vi "NMRFMTCP3.vi"() -> ()   [LabVIEW 2013]
uses:
  <vilib>/Analysis/2dsp.llb/Power Spectrum (DBL).vi
  <vilib>/Analysis/NI_AALBase.lvlib
  <vilib>/Analysis/NI_AALPro.lvlib
panel:
  out "Color Box":u32(colorbox)=16775210
  out "Measurement":enum16{"TEQ", "POL", "QCV"}(ring)
  in  "IP Address":string="192.168.0.4"
  out "FFT Vrms":dbl[](graph)=[0.015646766169154235, 0.0024982110948134676, 0.004931932619290262, 0.0008849248647205256, 0.002350996880382093, 0.0030163818070642833, 0.00321873871167239, 0.003596382576137373, 0.003663324666758867, 0.0009994820127704742, 0.0010747177604605467, 0.000922401354019206, 0.0012391697464639705, 0.0006999488109473508, 0.0009425280240178242, 0.0004953318625840751, 0.00024739643492388146, 0.00025317160361917977, 0.0006820660010904889, 0.0002670742831143547, 0.0002957484875645955, 0.00011731788024214158, 0.00015619144084108466, 7.076944387364928e-05, 0.00012524370826080074, 6.018279383692433e-05, 0.00024316035804602647, 0.00011417007815996506, 0.00010403858000381052, 4.3666360249968e-05, 8.722358525155538e-05, 6.472666110972202e-05, 7.949448204134939e-05, 4.547885976303066e-05, 3.653057660652789e-05, 9.501808066980672e-05, 2.9078658072371083e-05, 3.260626662558661e-05, 8.634700453978882e-05, 3.3459882147928455e-05, 8.341394425177981e-06, 8.711681853332232e-05, 6.11475957176423e-05, 4.284137586805631e-05, 4.7823392907281645e-06, 6.861730772494631e-05, 4.294940371852622e-05, 6.594416880768872e-05, 3.707630870344957e-05, 4.7322214771994784e-05, 8.140802356743123e-05, 4.401860468243618e-05, 6.432881992133859e-05, 7.158037542006712e-05, 5.347541272067149e-05, 1.0438009970739653e-05, 5.274129687041643e-05, 4.12553853761029e-05, 4.054935764826345e-05, 4.9349720124767846e-05, 2.4106567936024834e-05, 5.5044880104172067e-05, 6.473487682465393e-05, 1.8485431296046827e-05, 3.53153542517612e-05, 3.619008888621546e-05, 2.3642641556844984e-05, 1.9900497512436724e-05, 4.748254709029596e-05, 3.3152048109749e-05, 8.963711407032085e-06, 4.311995880312886e-05, 2.8267193875743532e-05, 1.7998716826374374e-05, 1.6139994180526443e-05, 6.40939445577451e-05, 3.5067385634575733e-05, 4.0420880711354366e-05, 2.7627165315509168e-05, 2.4593484558717827e-05, 1.625301397326756e-05, 1.58501158271677e-05, 4.3237292394627824e-05, 4.0973014105816716e-05, 2.8866404509190905e-05, 1.401615252343598e-05, 8.5877689760548e-06, 3.526207416355205e-05, 3.887541708076588e-05, 2.0945078547097e-05, 1.702451226539483e-05, 2.5281225738434016e-05, 1.5811372510805386e-05, 1.545238635589902e-05, 3.132846060147881e-05, 5.362881939741909e-05, 3.641158036427663e-05, 3.235440483664354e-05, 4.0993236124899505e-05, 3.337304052641068e-05, 5.448938806072747e-05, 5.448938806072747e-05, 3.337304052641068e-05, 4.0993236124899505e-05, 3.235440483664354e-05, 3.641158036427663e-05, 5.362881939741909e-05, 3.132846060147881e-05, 1.545238635589902e-05, 1.5811372510805386e-05, 2.5281225738434016e-05, 1.702451226539483e-05, 2.0945078547097e-05, 3.887541708076588e-05, 3.526207416355205e-05, 8.5877689760548e-06, 1.401615252343598e-05, 2.8866404509190905e-05, 4.0973014105816716e-05, 4.3237292394627824e-05, 1.58501158271677e-05, 1.625301397326756e-05, 2.4593484558717827e-05, 2.7627165315509168e-05, 4.0420880711354366e-05, 3.5067385634575733e-05, 6.40939445577451e-05, 1.6139994180526443e-05, 1.7998716826374374e-05, 2.8267193875743532e-05, 4.311995880312886e-05, 8.963711407032085e-06, 3.3152048109749e-05, 4.748254709029596e-05, 1.9900497512436724e-05, 2.3642641556844984e-05, 3.619008888621546e-05, 3.53153542517612e-05, 1.8485431296046827e-05, 6.473487682465393e-05, 5.5044880104172067e-05, 2.4106567936024834e-05, 4.9349720124767846e-05, 4.054935764826345e-05, 4.12553853761029e-05, 5.274129687041643e-05, 1.0438009970739653e-05, 5.347541272067149e-05, 7.158037542006712e-05, 6.432881992133859e-05, 4.401860468243618e-05, 8.140802356743123e-05, 4.7322214771994784e-05, 3.707630870344957e-05, 6.594416880768872e-05, 4.294940371852622e-05, 6.861730772494631e-05, 4.7823392907281645e-06, 4.284137586805631e-05, 6.11475957176423e-05, 8.711681853332232e-05, 8.341394425177981e-06, 3.3459882147928455e-05, 8.634700453978882e-05, 3.260626662558661e-05, 2.9078658072371083e-05, 9.501808066980672e-05, 3.653057660652789e-05, 4.547885976303066e-05, 7.949448204134939e-05, 6.472666110972202e-05, 8.722358525155538e-05, 4.3666360249968e-05, 0.00010403858000381052, 0.00011417007815996506, 0.00024316035804602647, 6.018279383692433e-05, 0.00012524370826080074, 7.076944387364928e-05, 0.00015619144084108466, 0.00011731788024214158, 0.0002957484875645955, 0.0002670742831143547, 0.0006820660010904889, 0.00025317160361917977, 0.00024739643492388146, 0.0004953318625840751, 0.0009425280240178242, 0.0006999488109473508, 0.0012391697464639705, 0.000922401354019206, 0.0010747177604605467, 0.0009994820127704742, 0.003663324666758867, 0.003596382576137373, 0.00321873871167239, 0.0030163818070642833, 0.002350996880382093, 0.0008849248647205256, 0.004931932619290262, 0.0024982110948134676]
  out "Raw NMR Graph / Ave":cluster{dbl, "Step Width (MHz)":dbl, dbl[][]}(graph)={212.47, "Step Width (MHz)"=0.0025, [[0.032, 0.031, 0.031, 0.031, 0.03, 0.03, 0.029, 0.029, 0.027, 0.027, 0.026, 0.025, 0.024, 0.023, 0.023, 0.023, 0.022, 0.021, 0.021, 0.021, 0.02, 0.02, 0.02, 0.019, 0.018, 0.017, 0.017, 0.016, 0.016, 0.015, 0.014, 0.014, 0.013, 0.013, 0.012, 0.012, 0.011, 0.011, 0.01, 0.009, 0.009, 0.009, 0.008, 0.008, 0.007, 0.007, 0.006, 0.006, 0.005, 0.005, 0.005, 0.005, 0.005, 0.004, 0.004, 0.004, 0.004, 0.003, 0.003, 0.002, 0.002, 0.002, 0.002, 0.002, 0.001, 0.0, 0.001, 0.001, -0.0, -0.0, -0.0, 0.0, 0.0, -0.0, -0.0, -0.0, -0.001, -0.0, -0.0, -0.0, -0.0, -0.0, 0.0, 0.001, 0.003, 0.004, 0.005, 0.007, 0.009, 0.011, 0.013, 0.016, 0.021, 0.026, 0.032, 0.039, 0.047, 0.054, 0.06, 0.061, 0.059, 0.054, 0.047, 0.038, 0.03, 0.023, 0.019, 0.015, 0.011, 0.008, 0.006, 0.005, 0.004, 0.003, 0.003, 0.003, 0.003, 0.003, 0.004, 0.006, 0.008, 0.01, 0.013, 0.016, 0.02, 0.025, 0.031, 0.037, 0.043, 0.047, 0.049, 0.049, 0.045, 0.038, 0.032, 0.026, 0.021, 0.016, 0.013, 0.009, 0.007, 0.006, 0.005, 0.004, 0.005, 0.005, 0.007, 0.009, 0.01, 0.013, 0.017, 0.021, 0.024, 0.026, 0.027, 0.026, 0.023, 0.02, 0.016, 0.013, 0.01, 0.008, 0.005, 0.004, 0.003, 0.003, 0.003, 0.003, 0.004, 0.005, 0.006, 0.008, 0.01, 0.013, 0.016, 0.018, 0.021, 0.022, 0.023, 0.023, 0.022, 0.021, 0.02, 0.019, 0.019, 0.017, 0.016, 0.014, 0.013, 0.012, 0.012, 0.012, 0.013, 0.014, 0.015, 0.018, 0.022, 0.026, 0.03, 0.035, 0.04], [0.03140634920634919, 0.03086031746031746, 0.030584126984126957, 0.0301301587301587, 0.029622222222222175, 0.029066666666666595, 0.028504761904761852, 0.027974603174603135, 0.02739047619047618, 0.0268095238095238, 0.026231746031746002, 0.02564126984126982, 0.025031746031746002, 0.02441269841269838, 0.023882539682539648, 0.023307936507936475, 0.0227269841269841, 0.02213650793650791, 0.021523809523809483, 0.020942857142857096, 0.020365079365079333, 0.01980317460317458, 0.019266666666666633, 0.018736507936507895, 0.01819047619047616, 0.01759682539682536, 0.01702857142857139, 0.016403174603174562, 0.015853968253968235, 0.015317460317460296, 0.014796825396825364, 0.014266666666666619, 0.013739682539682496, 0.013152380952380915, 0.012609523809523782, 0.012111111111111081, 0.011660317460317435, 0.011161904761904729, 0.010619047619047589, 0.010193650793650765, 0.00968888888888886, 0.009247619047619022, 0.008771428571428543, 0.008253968253968225, 0.007936507936507912, 0.00743174603174601, 0.006990476190476172, 0.006542857142857125, 0.0061142857142856945, 0.005711111111111095, 0.005276190476190463, 0.004882539682539673, 0.004539682539682529, 0.004184126984126974, 0.0038126984126984078, 0.0034603174603174613, 0.003066666666666669, 0.0027301587301587324, 0.002390476190476192, 0.0021015873015873027, 0.0017650793650793664, 0.0014476190476190485, 0.0011492063492063499, 0.0009174603174603177, 0.0007047619047619049, 0.0004952380952380952, 0.00022857142857142857, 3.1746031746029874e-06, -0.00013333333333333353, -0.00031428571428571454, -0.0004984126984126985, -0.000612698412698413, -0.0006952380952380956, -0.0007269841269841271, -0.0007746031746031748, -0.000758730158730159, -0.0006634920634920635, -0.0005492063492063494, -0.00037460317460317474, -0.0001333333333333334, 0.00021587301587301584, 0.0006126984126984127, 0.001111111111111112, 0.0017841269841269854, 0.002574603174603176, 0.0035968253968253947, 0.0047682539682539615, 0.006317460317460301, 0.00816507936507934, 0.010574603174603145, 0.013438095238095197, 0.016961904761904737, 0.021368253968253936, 0.026517460317460318, 0.032958730158730166, 0.03983174603174603, 0.0473174603174603, 0.054425396825396766, 0.059574603174603134, 0.06149523809523812, 0.05948253968253961, 0.053911111111111056, 0.046282539682539675, 0.037920634920634896, 0.03019682539682538, 0.023441269841269805, 0.018063492063492025, 0.01379047619047615, 0.010320634920634897, 0.007819047619047595, 0.005866666666666651, 0.004488888888888881, 0.0035650793650793653, 0.0029047619047619065, 0.0026444444444444462, 0.002625396825396827, 0.002949206349206351, 0.0036476190476190454, 0.004552380952380944, 0.0059238095238095066, 0.00776507936507934, 0.010101587301587271, 0.012961904761904728, 0.016565079365079338, 0.020765079365079327, 0.025907936507936477, 0.031787301587301545, 0.037806349206349205, 0.043555555555555535, 0.04799365079365076, 0.0500857142857143, 0.049082539682539665, 0.045193650793650765, 0.03926984126984125, 0.03255238095238093, 0.025993650793650763, 0.02026984126984124, 0.015615873015872984, 0.012006349206349177, 0.009222222222222194, 0.007247619047619024, 0.005873015873015858, 0.005019047619047606, 0.00465396825396824, 0.0048190476190476065, 0.005355555555555541, 0.006539682539682519, 0.008352380952380924, 0.010666666666666637, 0.013707936507936476, 0.016990476190476167, 0.020568253968253937, 0.02367936507936505, 0.02587619047619045, 0.026533333333333294, 0.02548888888888887, 0.022977777777777767, 0.019488888888888865, 0.015676190476190444, 0.012015873015872985, 0.008888888888888863, 0.0064412698412698215, 0.004644444444444433, 0.0033936507936507955, 0.0026476190476190493, 0.0023269841269841283, 0.0023682539682539695, 0.0027968253968253987, 0.0034666666666666682, 0.004488888888888881, 0.005847619047619032, 0.007587301587301563, 0.00974285714285711, 0.01238412698412695, 0.015180952380952366, 0.017987301587301552, 0.020568253968253947, 0.022244444444444414, 0.02298412698412696, 0.022806349206349177, 0.021958730158730122, 0.020914285714285673, 0.01988253968253965, 0.018968253968253926, 0.018088888888888863, 0.01697142857142854, 0.015765079365079336, 0.014476190476190452, 0.013276190476190433, 0.012355555555555535, 0.011892063492063456, 0.011822222222222185, 0.012349206349206322, 0.013492063492063461, 0.015085714285714256, 0.017514285714285687, 0.020606349206349173, 0.02439365079365076, 0.028895238095238068, 0.033825396825396835, 0.03893333333333329]]}
  in  "GPIB Addr (28)":refnum<visa-resource-name>="GPIB0::28::INSTR"
  out "Pedestal (V)":dbl=-0.0019038541666667472 format="%_2g"
  in  "Open Global Panel":bool=TRUE
  out "Peak center (MHz)":sgl=212.71716 format="%.3f"
  out "Telnet error out":errorcluster
  out "+3.3V supply":dbl=3.279 format="%_4g"
  out "Temp (C)":dbl=30.5 format="%_4g"
  out "RF OK":bool=TRUE
  out "Peak area (V-MHz)":sgl=3.3110082 format="%.5f"
  out "NMR Graph + Fit":cluster{cluster{dbl, "Numeric":dbl}[]}[](graph)=[{[{212.47, "Numeric"=0.0010780416666670367}, {212.4725, "Numeric"=0.0007280416666664439}, {212.475, "Numeric"=0.0013715416666658662}, {212.4775, "Numeric"=0.0020085416666652993}, {212.48, "Numeric"=0.001639041666664739}, {212.4825, "Numeric"=0.0022630416666642008}, {212.48499999999999, "Numeric"=0.001880541666663669}, {212.4875, "Numeric"=0.0024915416666700567}, {212.49, "Numeric"=0.001096041666669473}, {212.4925, "Numeric"=0.0016940416666689053}, {212.495, "Numeric"=0.001285541666668344}, {212.4975, "Numeric"=0.0008705416666678007}, {212.5, "Numeric"=0.00044904166666726465}, {212.5025, "Numeric"=2.1041666666739463e-05}, {212.505, "Numeric"=0.0005865416666662295}, {212.5075, "Numeric"=0.0011455416666657304}, {212.51, "Numeric"=0.0006980416666652412}, {212.5125, "Numeric"=0.0002440416666647698}, {212.515, "Numeric"=0.0007835416666643032}, {212.5175, "Numeric"=0.0013165416666698774}, {212.52, "Numeric"=0.0008430416666693587}, {212.5225, "Numeric"=0.0013630416666688587}, {212.525, "Numeric"=0.0018765416666683661}, {212.5275, "Numeric"=0.001383541666667887}, {212.53, "Numeric"=0.0008840416666674187}, {212.5325, "Numeric"=0.0003780416666669681}, {212.535, "Numeric"=0.0008655416666665259}, {212.5375, "Numeric"=0.0003465416666660901}, {212.54, "Numeric"=0.000821041666665673}, {212.5425, "Numeric"=0.00028904166666526235}, {212.545, "Numeric"=-0.0002494583333351322}, {212.54749999999999, "Numeric"=0.00020554166666448322}, {212.55, "Numeric"=-0.0003459583333308277}, {212.5525, "Numeric"=9.604166666873828e-05}, {212.555, "Numeric"=-0.000468458333331684}, {212.5575, "Numeric"=-3.945833333209459e-05}, {212.56, "Numeric"=-0.0006169583333324952}, {212.5625, "Numeric"=-0.0002009583333328806}, {212.565, "Numeric"=-0.0007914583333332561}, {212.5675, "Numeric"=-0.0013884583333336207}, {212.57, "Numeric"=-0.0009919583333339718}, {212.5725, "Numeric"=-0.0006019583333343103}, {212.575, "Numeric"=-0.001218458333334639}, {212.5775, "Numeric"=-0.000841458333334954}, {212.58, "Numeric"=-0.0014709583333310846}, {212.5825, "Numeric"=-0.0011069583333314509}, {212.585, "Numeric"=-0.0017494583333318063}, {212.5875, "Numeric"=-0.0013984583333321475}, {212.59, "Numeric"=-0.0020539583333324795}, {212.5925, "Numeric"=-0.0017159583333327972}, {212.595, "Numeric"=-0.0013844583333331058}, {212.5975, "Numeric"=-0.0010594583333334}, {212.6, "Numeric"=-0.0007409583333336843}, {212.6025, "Numeric"=-0.001428958333333957}, {212.605, "Numeric"=-0.001123458333334217}, {212.6075, "Numeric"=-0.0008244583333344643}, {212.60999999999999, "Numeric"=-0.0005319583333347018}, {212.6125, "Numeric"=-0.0012459583333317113}, {212.615, "Numeric"=-0.0009664583333319982}, {212.6175, "Numeric"=-0.0016934583333322725}, {212.62, "Numeric"=-0.001426958333332536}, {212.6225, "Numeric"=-0.0011669583333327868}, {212.625, "Numeric"=-0.0009134583333330268}, {212.6275, "Numeric"=-0.0006664583333332542}, {212.63, "Numeric"=-0.00142595833333347}, {212.6325, "Numeric"=-0.002191958333333673}, {212.635, "Numeric"=-0.0009644583333338654}, {212.6375, "Numeric"=-0.0007434583333340459}, {212.64, "Numeric"=-0.0015289583333342144}, {212.6425, "Numeric"=-0.001320958333332043}, {212.645, "Numeric"=-0.0011194583333322622}, {212.6475, "Numeric"=-0.0009244583333324688}, {212.65, "Numeric"=-0.0007359583333326637}, {212.6525, "Numeric"=-0.0005539583333328468}, {212.655, "Numeric"=-0.0003784583333330182}, {212.6575, "Numeric"=-0.00020945833333317794}, {212.66, "Numeric"=-0.001046958333333326}, {212.6625, "Numeric"=0.0001090416666665382}, {212.665, "Numeric"=0.0002585416666664143}, {212.6675, "Numeric"=0.0004015416666663021}, {212.67, "Numeric"=0.0005380416666662016}, {212.67249999999999, "Numeric"=0.0006680416666661128}, {212.675, "Numeric"=0.0007915416666674031}, {212.6775, "Numeric"=0.0019085416666672643}, {212.68, "Numeric"=0.004019041666667137}, {212.6825, "Numeric"=0.005123041666667022}, {212.685, "Numeric"=0.006220541666666918}, {212.6875, "Numeric"=0.008311541666666828}, {212.69, "Numeric"=0.010396041666666748}, {212.6925, "Numeric"=0.012474041666666678}, {212.695, "Numeric"=0.014545541666666623}, {212.6975, "Numeric"=0.017610541666666576}, {212.7, "Numeric"=0.022669041666666546}, {212.7025, "Numeric"=0.027721041666666522}, {212.705, "Numeric"=0.033766541666666997}, {212.7075, "Numeric"=0.040805541666666924}, {212.71, "Numeric"=0.048838041666666866}, {212.7125, "Numeric"=0.055864041666666815}, {212.715, "Numeric"=0.061883541666666785}, {212.7175, "Numeric"=0.06289654166666676}, {212.72, "Numeric"=0.06090304166666675}, {212.7225, "Numeric"=0.05590304166666675}, {212.725, "Numeric"=0.04889654166666676}, {212.7275, "Numeric"=0.039883541666666786}, {212.73, "Numeric"=0.03186404166666682}, {212.7325, "Numeric"=0.024838041666666866}, {212.73499999999999, "Numeric"=0.020805541666666923}, {212.7375, "Numeric"=0.016766541666666517}, {212.74, "Numeric"=0.012721041666666526}, {212.7425, "Numeric"=0.009669041666666546}, {212.745, "Numeric"=0.007610541666666579}, {212.7475, "Numeric"=0.006545541666666623}, {212.75, "Numeric"=0.005474041666666679}, {212.7525, "Numeric"=0.004396041666666748}, {212.755, "Numeric"=0.004311541666666827}, {212.7575, "Numeric"=0.004220541666666919}, {212.76, "Numeric"=0.004123041666667022}, {212.7625, "Numeric"=0.004019041666667137}, {212.765, "Numeric"=0.004908541666667265}, {212.7675, "Numeric"=0.006791541666666036}, {212.77, "Numeric"=0.008668041666666113}, {212.7725, "Numeric"=0.010538041666666203}, {212.775, "Numeric"=0.013401541666666301}, {212.7775, "Numeric"=0.016258541666666414}, {212.78, "Numeric"=0.02010904166666654}, {212.7825, "Numeric"=0.024953041666666675}, {212.785, "Numeric"=0.03079054166666682}, {212.7875, "Numeric"=0.03662154166666698}, {212.79, "Numeric"=0.04244604166666715}, {212.7925, "Numeric"=0.04626404166666734}, {212.795, "Numeric"=0.04807554166666753}, {212.79749999999999, "Numeric"=0.04788054166666774}, {212.8, "Numeric"=0.04367904166666563}, {212.8025, "Numeric"=0.03647104166666578}, {212.805, "Numeric"=0.030256541666665953}, {212.8075, "Numeric"=0.024035541666666133}, {212.81, "Numeric"=0.018808041666666327}, {212.8125, "Numeric"=0.01357404166666653}, {212.815, "Numeric"=0.010333541666666744}, {212.8175, "Numeric"=0.0060865416666669725}, {212.82, "Numeric"=0.0038330416666672133}, {212.8225, "Numeric"=0.002573041666667464}, {212.825, "Numeric"=0.0013065416666677276}, {212.8275, "Numeric"=3.354166666800183e-05}, {212.83, "Numeric"=0.0007540416666650743}, {212.8325, "Numeric"=0.00046804166666529826}, {212.835, "Numeric"=0.0021755416666655357}, {212.8375, "Numeric"=0.0038765416666657823}, {212.84, "Numeric"=0.004571041666666043}, {212.8425, "Numeric"=0.007259041666666315}, {212.845, "Numeric"=0.010940541666666602}, {212.8475, "Numeric"=0.014615541666666895}, {212.85, "Numeric"=0.017284041666667204}, {212.8525, "Numeric"=0.018946041666667517}, {212.855, "Numeric"=0.019601541666667853}, {212.8575, "Numeric"=0.01825054166666819}, {212.85999999999999, "Numeric"=0.01489304166666855}, {212.8625, "Numeric"=0.011529041666664741}, {212.865, "Numeric"=0.007158541666665046}, {212.8675, "Numeric"=0.0037815416666653603}, {212.87, "Numeric"=0.00039804166666569055}, {212.8725, "Numeric"=-0.001991958333333971}, {212.875, "Numeric"=-0.00538845833333362}, {212.8775, "Numeric"=-0.006791458333333256}, {212.88, "Numeric"=-0.00820095833333288}, {212.8825, "Numeric"=-0.008616958333332495}, {212.885, "Numeric"=-0.009039458333332095}, {212.8875, "Numeric"=-0.009468458333331684}, {212.89, "Numeric"=-0.008903958333331262}, {212.8925, "Numeric"=-0.00834595833333589}, {212.895, "Numeric"=-0.007794458333335517}, {212.8975, "Numeric"=-0.006249458333335132}, {212.9, "Numeric"=-0.004710958333334737}, {212.9025, "Numeric"=-0.002178958333334328}, {212.905, "Numeric"=0.0003465416666660901}, {212.9075, "Numeric"=0.0018655416666665233}, {212.91, "Numeric"=0.004378041666666968}, {212.9125, "Numeric"=0.004884041666667419}, {212.915, "Numeric"=0.005383541666667887}, {212.9175, "Numeric"=0.004876541666668365}, {212.92, "Numeric"=0.003363041666668857}, {212.92249999999999, "Numeric"=0.0018430416666693596}, {212.925, "Numeric"=0.00031654166666385004}, {212.9275, "Numeric"=-0.0012164583333356986}, {212.93, "Numeric"=-0.001755958333335232}, {212.9325, "Numeric"=-0.004301958333334756}, {212.935, "Numeric"=-0.005854458333334269}, {212.9375, "Numeric"=-0.008413458333333769}, {212.94, "Numeric"=-0.00997895833333326}, {212.9425, "Numeric"=-0.011550958333332736}, {212.945, "Numeric"=-0.012129458333332201}, {212.9475, "Numeric"=-0.012714458333331655}, {212.95, "Numeric"=-0.012305958333331094}, {212.9525, "Numeric"=-0.011903958333330526}, {212.955, "Numeric"=-0.011508458333336854}, {212.9575, "Numeric"=-0.009119458333336335}, {212.96, "Numeric"=-0.005736958333335799}, {212.9625, "Numeric"=-0.002360958333335261}, {212.965, "Numeric"=0.0010085416666652984}, {212.9675, "Numeric"=0.00537154166666587}, {212.97, "Numeric"=0.009728041666666444}]}]
  out "# Good Spectra":i32=989
  out "Pedestal OK":bool=TRUE
  out "Sweep #":i32=316
  out "1st Sweep":bool
  out "ADC volts OK":bool=TRUE
  out "Peak Height Distribution":cluster{"Y":dbl[], "Y":dbl[]}[](graph)=[{"Y"=[0.06173175000000009, 0.061768833333333426, 0.06180591666666676, 0.06184300000000009, 0.061880083333333426, 0.06191716666666676, 0.06195425000000009, 0.061991333333333426, 0.06202841666666676, 0.06206550000000009, 0.062102583333333426, 0.06213966666666676, 0.06217675000000009, 0.062213833333333426, 0.06225091666666676, 0.06228800000000009, 0.06232508333333343, 0.06236216666666676, 0.062399250000000094, 0.06243633333333343, 0.06247341666666676, 0.0625105000000001, 0.06254758333333343, 0.06258466666666676, 0.0626217500000001, 0.06265883333333343, 0.06269591666666677, 0.0627330000000001, 0.06277008333333343, 0.06280716666666676, 0.0628442500000001, 0.06288133333333343, 0.06291841666666677, 0.0629555000000001, 0.06299258333333344, 0.06302966666666676, 0.0630667500000001, 0.06310383333333343, 0.06314091666666677, 0.0631780000000001, 0.06321508333333344, 0.06325216666666676, 0.0632892500000001, 0.06332633333333343, 0.06336341666666677, 0.0634005000000001, 0.06343758333333344, 0.06347466666666676, 0.0635117500000001, 0.06354883333333343, 0.06358591666666677, 0.0636230000000001, 0.06366008333333342, 0.06369716666666676, 0.06373425000000009, 0.06377133333333343, 0.06380841666666676, 0.0638455000000001, 0.06388258333333342, 0.06391966666666676, 0.06395675000000009, 0.06399383333333343, 0.06403091666666676, 0.0640680000000001, 0.06410508333333342, 0.06414216666666676, 0.06417925000000009, 0.06421633333333343, 0.06425341666666676, 0.0642905000000001, 0.06432758333333342, 0.06436466666666676, 0.06440175000000009, 0.06443883333333343, 0.06447591666666676, 0.0645130000000001, 0.06455008333333342, 0.06458716666666676, 0.06462425000000009, 0.06466133333333343, 0.06469841666666676, 0.0647355000000001, 0.06477258333333342, 0.06480966666666677, 0.06484675000000009, 0.06488383333333343, 0.06492091666666676, 0.0649580000000001, 0.06499508333333343, 0.06503216666666677, 0.06506925000000009, 0.06510633333333343, 0.06514341666666676, 0.0651805000000001, 0.06521758333333343, 0.06525466666666677, 0.06529175000000009, 0.06532883333333343, 0.06536591666666676, 0.0654030000000001], "Y"=[1.0, 0.0, 1.0, 2.0, 2.0, 3.0, 2.0, 0.0, 3.0, 4.0, 2.0, 8.0, 6.0, 8.0, 2.0, 6.0, 4.0, 4.0, 5.0, 9.0, 6.0, 8.0, 10.0, 8.0, 7.0, 8.0, 12.0, 10.0, 10.0, 16.0, 10.0, 18.0, 13.0, 6.0, 15.0, 17.0, 17.0, 16.0, 17.0, 14.0, 19.0, 17.0, 13.0, 16.0, 23.0, 22.0, 22.0, 16.0, 26.0, 21.0, 24.0, 17.0, 19.0, 18.0, 13.0, 24.0, 18.0, 18.0, 22.0, 17.0, 17.0, 8.0, 14.0, 14.0, 14.0, 11.0, 18.0, 22.0, 16.0, 10.0, 15.0, 16.0, 8.0, 10.0, 15.0, 9.0, 3.0, 4.0, 6.0, 8.0, 7.0, 5.0, 7.0, 3.0, 6.0, 4.0, 5.0, 4.0, 4.0, 0.0, 2.0, 0.0, 1.0, 1.0, 0.0, 2.0, 1.0, 2.0, 1.0, 1.0]}]
  out "S/N":dbl=88.94507757693563 format="%_3g"
  out "Peak mean (V)":dbl=0.06354517665149992 format="%_4g"
  out "Pedestal Diff (V)":sgl=-0.00015841666 format="%.3f"
  out "Peak amp (V)":sgl=0.06289654 format="%.3f"
  out "SMT error out":errorcluster
  out "Peak RMS (mV)":dbl=0.7144316288502269 format="%.3f"
  # "E1039 NMR Panel"
  # "Results"
  # "A\nv\ne\nr\na\ng\ne\ns"
  # "S\nw\ne\ne\np"
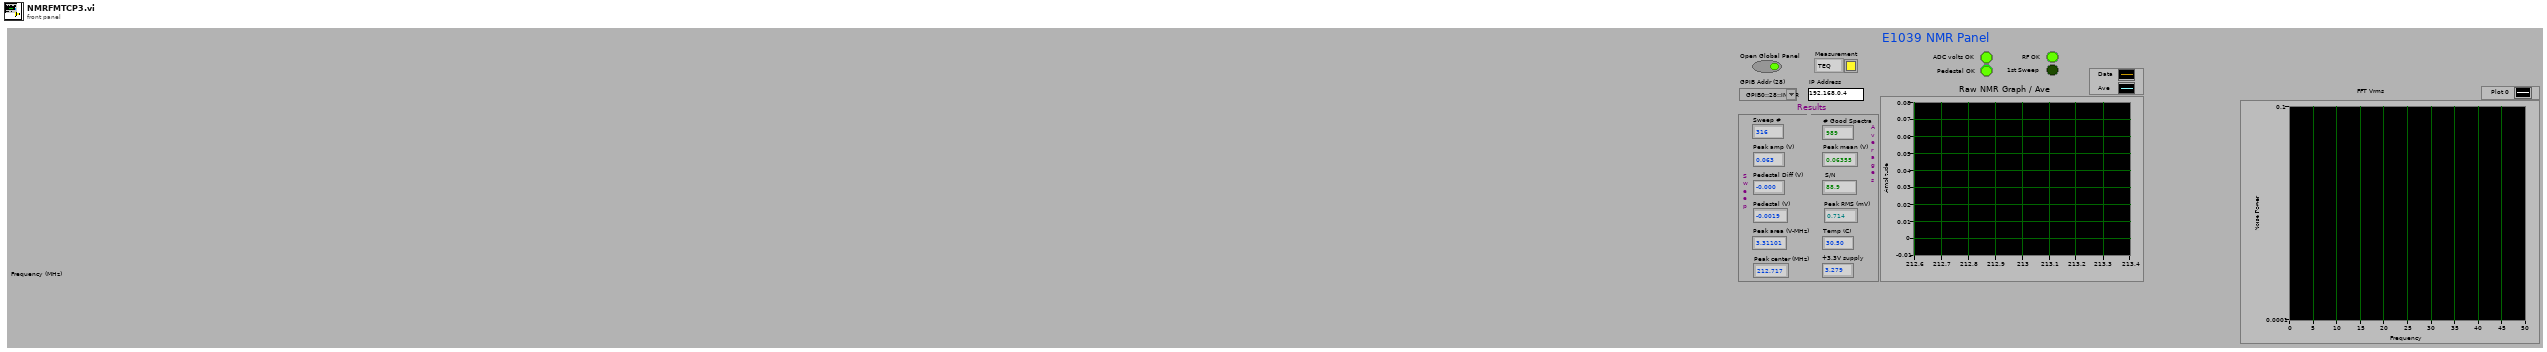
[diagram p1: front panel]
types:
  T1 = enum32{"Invalid", "Standard", "Closed", "Hidden", "Minimized", "Maximized"}
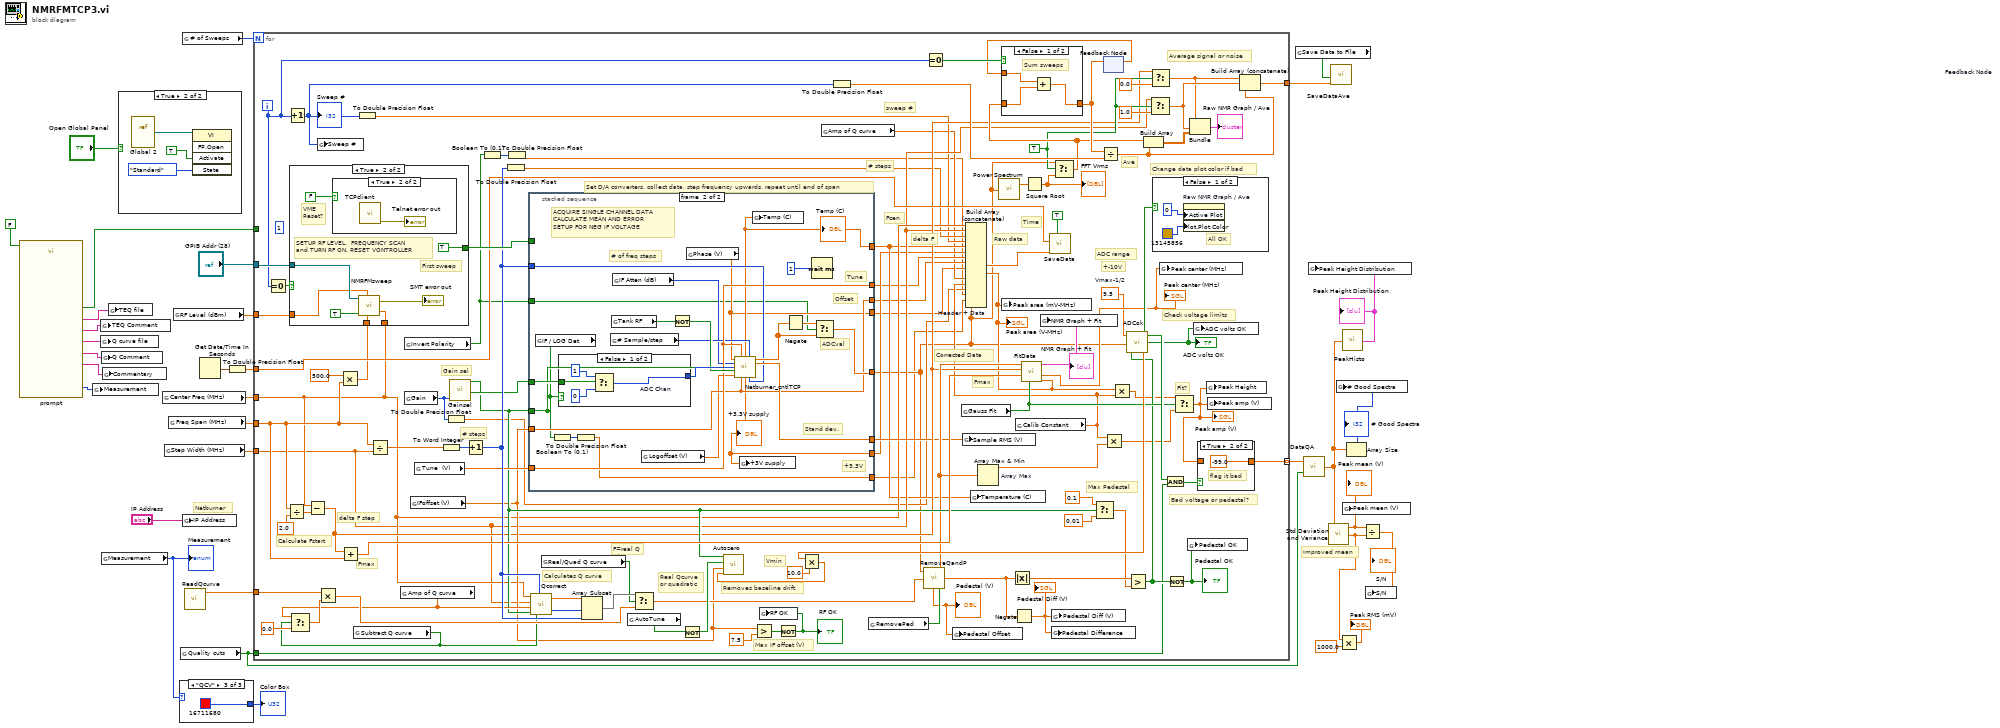
[diagram p0: block diagram]
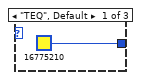
[diagram p2: hidden frame]
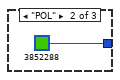
[diagram p3: hidden frame]
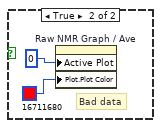
[diagram p6: hidden frame]
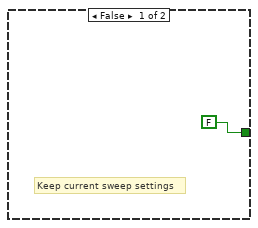
[diagram p8: hidden frame]
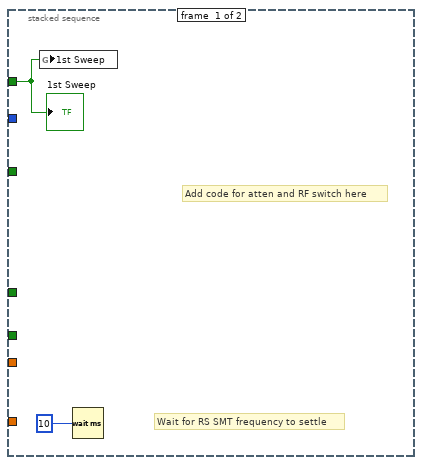
[diagram p10: hidden frame]
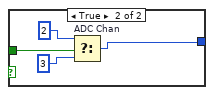
[diagram p11: hidden frame]
diagram:
  # "Netburner"
  # "Improved mean"
  n1 = call "prompt.vi"("Enable"=FALSE) -> ("Measurement"=w2:enum16{"TEQ", "POL", "QCV"}, "Run comment"=w3:string, "Q curve comment"=w4:string, "Q curve file"=w5:string, "TE Comment"=w6:string, "TE peak file"=w7:string, "OK"=w8:bool)  [unwired: 11 in, 1 out]
  n2 = global write "Global 2.vi" "Measurement"(w2) -> ()
  n3 = global write "Global 2.vi" "TEQ Comment"(w6) -> ()
  n4 = global write "Global 2.vi" "Q curve file"(w5) -> ()
  n5 = global write "Global 2.vi" "Q Comment"(w4) -> ()
  n6 = global read "Global 2.vi" "Measurement"() -> (w10:enum16{"TEQ", "POL", "QCV"})
  "Measurement" <- w10
  n7 = global write "Global 2.vi" "Commentary"(w3) -> ()
  n8 = global write "Global 2.vi" "TEQ file"(w7) -> ()
  n9 = case shown="True" "Open Global Panel" {
    frame False {
    }
    frame True {
      n10 = vi-ref "Global 2.vi"() -> (w36:refnum<vi>)
      n11 = invoke class="VI" method="FP.Open"(reference=w36, "Activate"=TRUE, "State"=T1."Standard") -> ()  [unwired: 2 in, 5 out]
    }
  }
  n12 = global read "Global 2.vi" "Center Freq (MHz)"() -> (w28:dbl)
  n13 = global read "Global 2.vi" "Step Width (MHz)"() -> (w26:dbl)
  n14 = global read "Global 2.vi" "Freq Span (MHz)"() -> (w27:dbl)
  n15 = global read "Global 2.vi" "RF Level (dBm)"() -> (w29:dbl)
  n16 = case shown="\"QCV\"" w10 {
    tunnel: [u32 16775210 ("Color Box 2") u32 3852288 ("Color Box 2") u32 16711680 ("Color Box 2")] -> w9
    frame "TEQ", Default {
    }
    frame "POL" {
    }
    frame "QCV" {
    }
  }
  "Color Box" <- w9
  n17 = global read "Global 2.vi" "Quality cuts"() -> (w25:bool)
  n18 = global write "Global 2.vi" "IP Address"("IP Address") -> ()
  n19 = global read "Global 2.vi" "# of Sweeps"() -> (w30:i32)
  n20 = call "ReadQcurve.vi"() -> ("Array"=w15:dbl[])  [unwired: 2 in]
  n21 = Get Date/Time In Seconds() -> (seconds since 1Jan1904=w31:timestamp)
  n22 = To Double Precision Float(number=w31) -> (double precision float=w16:dbl)
  n23 = for {
    N: w30 -> [_]
    tunnel: [w133] -> w33 mode=indexing
    tunnel: w25 -> [w93]
    tunnel: w28 -> [w61]
    tunnel: w27 -> [w74]
    tunnel: w26 -> [w60]
    tunnel: "GPIB Addr (28)" -> [w128]
    tunnel: w29 -> [w127]
    tunnel: w16 -> [w126]
    tunnel: w15 -> [w118]
    tunnel: [w80] -> w18
    tunnel: w8 -> [_]
    i -> [w76]
    (unwired) 1
    w66 = TRUE
    w87 = 9.5  # Vmax-1/2
    # "Average signal or noise"
    # "Check voltage limits"
    # "Ave"
    # "Max Pedestal"
    # "Gain sel"
    # "F=real Q"
    # "Real Qcurve\nor quadratic"
    # "+-10V"
    # "Change data plot color if bad"
    # "Max IF offset (V)"
    # "Fmax"
    # "Fit?"
    # "Fmax"
    # "Time"
    # "Vmin"
    # "Raw data"
    # "Corrected Data"
    # "Fcen"
    # "delta F"
    # "# steps"
    # "ADC range"
    # "sweep #"
    # "Set D/A converters, collect data, step frequency upwards, repeat until end of span"
    # "Calculates Q curve"
    # "Removes baseline drift"
    # "Bad voltage or pedestal?"
    # "# steps"
    # "Calculate Fstart"
    # "delta F step"
    n24 = Equal To 0?(x=w76) -> (x = 0?=w135:bool)
    n25 = Divide(x=w74, y=sgl 2.0) -> (x/y=w139:dbl)
    n26 = Increment(x=w76) -> (x+1=w91:i32)
    "Sweep #" <- w91
    n27 = Subtract(x=w61, y=w139) -> (x-y=w64:dbl)
    n28 = global write "Global 2.vi" "Sweep #"(w91) -> ()
    n29 = Multiply(x=500.0, y=w74) -> (x*y=w73:dbl)
    n30 = case shown="True" w135 {
      tunnel: w61 -> [_ w159]
      tunnel: w73 -> [_ w160]
      tunnel: [FALSE TRUE] -> w134
      tunnel: w128 -> [_ w156]
      tunnel: w127 -> [_ w155]
      frame False {
        # "Keep current sweep settings"
      }
      frame True {
        # "VME\nReset?"
        # "First sweep"
        # "SETUP RF LEVEL,  FREQUENCY SCAN\nand TURN RF ON. RESET VONTROLLER"
        n31 = case shown="True" FALSE {
          frame False {
          }
          frame True {
            n32 = call "TCPclient.vi"() -> ("Telnet error"=→"Telnet error out":errorcluster)  [unwired: 4 in, 3 out]
          }
        }
        n33 = call "NMRFMsweep.vi"("Center Freq (MHz)"=w159, "Freq Span (kHz)"=w160, "RF Level (dBm)"=w155, "Program"=TRUE, "GPIB Addr (28)"=w156) -> ("error out"=→"SMT error out":errorcluster)  [unwired: 2 in]
      }
    }
    n34 = Add(x=w64, y=w74) -> (x+y=w123:dbl)
    n35 = global read "Global 2.vi" "Subtract Q curve"() -> (w109:bool)
    n36 = To Double Precision Float(number=w91) -> (double precision float=w58:dbl)
    n37 = Divide(x=w74, y=w60) -> (x/y=w141:dbl)
    n38 = global read "Global 2.vi" "Amp of Q curve"() -> (w110:dbl)
    n39 = Select(t=w110, s=w109, f=0.0) -> (s? t:f=w115:dbl)
    n40 = Multiply(x=w118, y=w115) -> (x*y=w117:dbl[])
    n41 = global read "Global 2.vi" "Invert Polarity"() -> (w42:bool)
    n42 = global read "Global 2.vi" "Gain"() -> (w47:enum16{"LOW", "HI", "MAX"})
    n43 = global read "Global 2.vi" "IFoffset (V)"() -> (w79:dbl)
    n44 = global read "Global 2.vi" "Tune  (V)"() -> (w111:dbl)
    n45 = To Word Integer(number=w141) -> (16bit integer=w138:i16)
    n46 = To Double Precision Float(number=w47) -> (double precision float=w46:dbl)
    n47 = call "Gainsel.vi"("Gain"=w47) -> ("LO"=w83:bool, "MAX"=w82:bool)  [unwired: 1 out]
    n48 = Increment(x=w138) -> (x+1=w129:i16)
    n49 = Boolean To (0,1)(Boolean=w42) -> (0, 1=w43:i16)
    n50 = To Double Precision Float(number=w129) -> (double precision float=w59:dbl)
    n51 = To Double Precision Float(number=w43) -> (double precision float=w41:dbl)
    n52 = stacked-sequence {
      tunnel: [_ w181] -> w62
      tunnel: [_ w185] -> w45
      tunnel: w129 -> [_ w179]
      tunnel: w79 -> [_ w176]
      tunnel: w83 -> [_ w183]
      tunnel: w134 -> [w162 _]
      tunnel: w111 -> [_ w177]
      tunnel: [_ w170] -> w57
      tunnel: [_ w169] -> w56
      tunnel: [_ w177] -> w55
      tunnel: [_ w176] -> w54
      tunnel: [_ w175] -> _
      tunnel: w82 -> [_ w175]
      tunnel: [_ w168] -> w44
      tunnel: w42 -> [_ w167]
      tunnel: [_ w164] -> w40
      frame #0 {
        # "Add code for atten and RF switch here"
        # "Wait for RS SMT frequency to settle"
        n53 = global write "Global 2.vi" "1st Sweep"(w162) -> ()
        n54 = Wait (ms)(milliseconds to wait=10) -> ()  [unwired: 1 out]
        "1st Sweep" <- w162
      }
      frame #1 {
        # "+3.3V"
        # "Offset"
        # "Tune"
        # "Stand dev."
        # "ADCval"
        # "ACQUIRE SINGLE CHANNEL DATA\nCALCULATE MEAN AND ERROR\nSETUP FOR NEG IF VOLTAGE"
        # "# of freq steps"
        n55 = global read "Global 2.vi" "IF / LOG Det"() -> (w166:bool)
        n56 = Boolean To (0,1)(Boolean=w166) -> (0, 1=w165:i16)
        n57 = case shown="False" w166 {
          tunnel: w183 -> [w190 w191]
          tunnel: [w187 w192] -> w180
          frame False {
            n58 = Select "ADC Chan"(t=1, s=w190, f=0) -> (s? t:f=w187:i32)
          }
          frame True {
            n59 = Select "ADC Chan"(t=2, s=w191, f=3) -> (s? t:f=w192:i32)
          }
        }
        n60 = To Double Precision Float(number=w165) -> (double precision float=w164:dbl)
        n61 = global read "Global 2.vi" "# Sample/step"() -> (w172:i32)
        n62 = global read "Global 2.vi" "Tank RF"() -> (w173:bool)
        n63 = global read "Global 2.vi" "IF Atten (dB)"() -> (w171:i8)
        n64 = global read "Global 2.vi" "Logoffset (V)"() -> (w174:dbl)
        n65 = Not(x=w173) -> (.not. x?=w178:bool)
        n66 = global read "Global 2.vi" "Phase (V)"() -> (w168:dbl)
        n67 = call "Netburner_cntlTCP.vi"("Phase Volt"=w168, "Tune Volt"=w177, "# Data"=w172, "IF Atten (dB)"=w171, "NMR ADC"=w180, "Hi Gain"=w175, "Tank RF"=w178, "LogOff Volt"=w174, "IFOff Volt"=w176, "# f steps"=w179) -> ("Temp (C)"=w170:dbl, "ADC value"=w182:dbl[], "ADC Std Dev"=w181:dbl, "Volts"=w169:dbl)  [unwired: 2 out]
        "Temp (C)" <- w170
        "+3.3V supply" <- w169
        n68 = global write "Global 2.vi" "+3V supply"(w169) -> ()
        n69 = global write "Global 2.vi" "Temp (C)"(w170) -> ()
        n70 = Negate(x=w182) -> (-x=w184:dbl[])
        n71 = Wait (ms)(milliseconds to wait=1) -> ()  [unwired: 1 out]
        n72 = Select(t=w184, s=w167, f=w182) -> (s? t:f=w185:dbl[])
      }
    }
    n73 = call "Qcorrect.vi"("Subtract Q curve"=w109, "Nstep"=w129, "Max Gain"=w82, "Amp of Q curve"=w110, "Step Width (MHz)"=w60, "Center Freq (MHz)"=w61) -> ("Start"=w136:i32, "Array"=w137:dbl[])
    n74 = global read "Global 2.vi" "Real/Quad Q curve"() -> (w108:bool)
    n75 = Array Subset "Array Subset"(array=w137, index=w136, length=w129) -> (w120:dbl[])
    n76 = global read "Global 2.vi" "AutoTune"() -> (w106:bool)
    n77 = Select(t=w120, s=w108, f=w117) -> (s? t:f=w119:dbl[])
    n78 = Not(x=w106) -> (.not. x?=w121:bool)
    n79 = Greater?(x=w79, y=7.5) -> (0:w124:bool)
    n80 = Not(x=w124) -> (.not. x?=w102:bool)
    "RF OK" <- w102
    n81 = global write "Global 2.vi" "RF OK"(w102) -> ()
    n82 = global read "Global 2.vi" "Amp of Q curve"() -> (w49:dbl)
    n83 = To Double Precision Float(number=w91) -> (double precision float=w85:dbl)
    n84 = global read "Global 2.vi" "RemovePed"() -> (w107:bool)
    n85 = call "RemoveQandP.vi"("Subtract Ped?"=w107, "Qcurve"=w119, "Raw data"=w45) -> ("Ped L-R"=w130:dbl, "Corrected data"=w70:dbl[], "Ped Offfset"=w97:dbl)
    "Pedestal (V)" <- w97
    n86 = Equal To 0?(x=w76) -> (x = 0?=w90:bool)
    n87 = global write "Global 2.vi" "Pedestal Offset"(w97) -> ()
    n88 = global read "Global 2.vi" "Gauss Fit"() -> (w105:bool)
    n89 = global write "Global 2.vi" "Sample RMS (V)"(w62) -> ()
    n90 = global write "Global 2.vi" "Temperature (C)"(w57) -> ()
    n91 = Array Max & Min "Array Max"(array=w70) -> (max value=w53:dbl)  [unwired: 3 out]
    n92 = call-poly <vilib>:"Power Spectrum.vi"("X"=w45) -> ("Power Spectrum"=w75:dbl[])  [unwired: 1 out]
    n93 = Absolute Value ("Abs Value")(x=w130) -> (abs(x)=w131:dbl)
    n94 = Negate(x=w130) -> (-x=w98:dbl)
    "Pedestal Diff (V)" <- w98
    n95 = global read "Global 2.vi" "Calib Constant"() -> (w48:dbl)
    n96 = call "FitData.vi"("Fit?"=w105, "Fmax"=w123, "Fmin"=w64, "Yarray"=w70) -> ("Peak Area (mV-MHz)"=w51:dbl, "Center Freq (MHz)"=w101:dbl, "NMR Graph + Fit"=w99:cluster{cluster{dbl, "Numeric":dbl}[]}[])  [unwired: 2 out]
    "NMR Graph + Fit" <- w99
    "Peak area (V-MHz)" <- w51
    "Peak center (MHz)" <- w101
    n97 = Build Array (concatenate) "Header + Data"(w61, w60, w59, w58, w57, w56, w55, w54, w44, w51, w49, w48, w46, w41, w40, w45) -> (w77:dbl[])
    n98 = global write "Global 2.vi" "Peak area (mV-MHz)"(w51) -> ()
    n99 = Square Root(x=w75) -> (sqrt(x)=w71:dbl[])
    "FFT Vrms" <- w71
    n100 = global write "Global 2.vi" "NMR Graph + Fit"(w99) -> ()
    n101 = call "SaveData.vi"("Array"=w77, "Save Data to File"=TRUE, "Ext time (sec)"=w126) -> ()  [unwired: 1 out]
    n102 = global write "Global 2.vi" "Pedestal Difference"(w98) -> ()
    n103 = global write "Global 2.vi" "Pedestal Diff (V)"(w98) -> ()
    n104 = Select(t=w45, s=w66, f=w71) -> (s? t:f=w69:dbl[])
    n105 = Select(t=0.1, s=w82, f=0.01) -> (s? t:f=w92:dbl)
    n106 = feedback #1 "Feedback Node"() -> (w89:dbl[])  [unwired: 1 in]
    n107 = case shown="False" w90 {
      tunnel: w69 -> [w143 w145]
      tunnel: [w142 w145] -> w86
      tunnel: w89 -> [w144 _]
      frame False {
        # "Sum sweeps"
        n108 = Add(x=w144, y=w143) -> (x+y=w142:dbl[])
      }
      frame True {
        # "Initialize"
      }
    }
    n109 = Divide(x=w86, y=w85) -> (x/y=w81:dbl[])
    n110 = feedback-in #1(w86) -> ()
    n111 = Multiply(x=w48, y=w53) -> (x*y=w52:dbl)
    n112 = Multiply(x=w51, y=w48) -> (x*y=w50:dbl)
    n113 = Greater?(x=w131, y=w92) -> (0:w94:bool)
    n114 = call "ADCok.vi"("PedOK"=w94, "Array"=w45, "Vmax-1/2"=w87) -> ("Vmin"=w114:dbl, "ADC voltages OK"=w104:bool, "Allok"=w122:bool)
    "ADC volts OK" <- w104
    n115 = Multiply(x=w114, y=10.0) -> (x*y=w112:dbl)
    n116 = call "Autozero.vi"("Vmin (V)"=w112, "IFoffset (V)"=w79, "Enable"=w121, "Max Gain"=w82) -> ()
    n117 = Build Array "Build Array"(w69, w81) -> (w84:dbl[][])
    n118 = Select(t=w60, s=w66, f=1.0) -> (s? t:f=w67:dbl)
    n119 = Select(t=w64, s=w66, f=0.0) -> (s? t:f=w63:dbl)
    n120 = case shown="False" w122 {
      frame False {
        # "All OK"
        n121 = property on="Raw NMR Graph / Ave" class="WFGraph (strict)"("Active Plot"=0, "Plot.Plot Color"=u32 13145856) -> ()  [unwired: 2 in, 2 out]
      }
      frame True {
        # "Bad data"
        n122 = property on="Raw NMR Graph / Ave" class="WFGraph (strict)"("Active Plot"=0, "Plot.Plot Color"=u32 16711680) -> ()  [unwired: 2 in, 2 out]
      }
    }
    n123 = global write "Global 2.vi" "Peak center (MHz)"(w101) -> ()
    n124 = And(x=w122, y=w93) -> (x .and. y?=w132:bool)
    n125 = Not(x=w94) -> (.not. x?=w103:bool)
    "Pedestal OK" <- w103
    n126 = Select(t=w50, s=w105, f=w52) -> (s? t:f=w100:dbl)
    "Peak amp (V)" <- w100
    n127 = global write "Global 2.vi" "Pedestal OK"(w103) -> ()
    n128 = Bundle(w63, "Step Width (MHz)"=w67, w84) -> (→"Raw NMR Graph / Ave":cluster{dbl, "Step Width (MHz)":dbl, dbl[][]})  [unwired: 1 in]
    n129 = global write "Global 2.vi" "ADC volts OK"(w104) -> ()
    n130 = case shown="True" w132 {
      tunnel: [w150 -99.0] -> w133
      tunnel: w100 -> [w150 _]
      frame False {
        # "Data OK"
      }
      frame True {
        # "flag it bad"
      }
    }
    n131 = global write "Global 2.vi" "Peak Height"(w100) -> ()
    n132 = global write "Global 2.vi" "Peak amp (V)"(w100) -> ()
    n133 = Build Array (concatenate) "Build Array"(w63, w67, w81) -> (w80:dbl[])
  }
  n134 = global read "Global 2.vi" "Save Data to File"() -> (w17:bool)
  n135 = call "DataQA.vi"("Quality cuts"=w25, "Data In"=w33) -> ("Data Out"=w32:dbl[])
  n136 = call <vilib>:"Std Deviation and Variance.vi"("X"=w32) -> ("mean"=w23:dbl, "standard deviation"=w12:dbl)  [unwired: 1 in, 1 out]
  "Peak mean (V)" <- w23
  n137 = call "SaveDataAve.vi"("Array"=w18, "Save Data to File"=w17) -> ()  [unwired: 1 in, 1 out]
  n138 = Multiply(x=w12, y=1000.0) -> (x*y=→"Peak RMS (mV)":dbl)
  n139 = call "PeakHisto.vi"("Data Out"=w32) -> ("XY Graph"=w21:cluster{"Y":dbl[], "Y":dbl[]}[])
  "Peak Height Distribution" <- w21
  n140 = global write "Global 2.vi" "Peak Height Distribution"(w21) -> ()
  n141 = global write "Global 2.vi" "Peak mean (V)"(w23) -> ()
  n142 = Array Size(array=w32) -> (size(s)=w22:i32)
  "# Good Spectra" <- w22
  n143 = global write "Global 2.vi" "# Good Spectra"(w22) -> ()
  n144 = Divide(x=w23, y=w12) -> (x/y=w24:dbl)
  "S/N" <- w24
  n145 = global write "Global 2.vi" "S/N"(w24) -> ()
